vi "ColourElementTree(SubVI).vi"(8 "Error In":errorcluster, 9 "Color":u32(colorbox), 10 "SR Number":string, 11 "TreeControl in":refnum<vi>) -> (0 "Error Out":errorcluster)   [LabVIEW 2017, in "DS_Lib.lvlib" / "SRReportParser.lvlib"]
uses:
  SRReportParser.lvlib
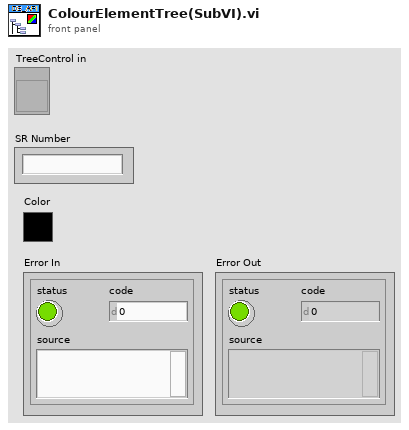
[diagram p1: front panel]
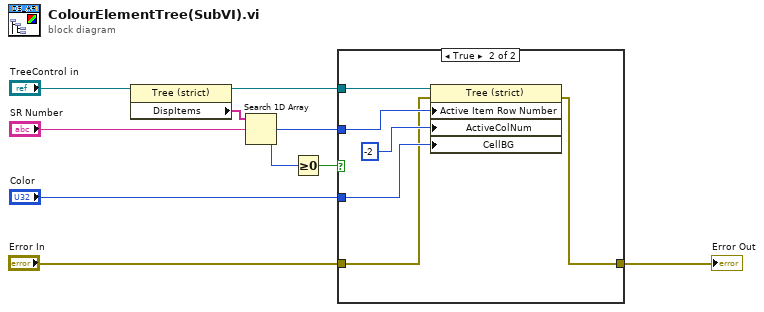
[diagram p0: block diagram]
diagram:
  n1 = property class="Tree (strict)"(reference="TreeControl in") -> (reference out=w9:refnum<vi>, "DispItems"=w8:string[])  [unwired: 1 in, 1 out]
  n2 = Search 1D Array(1D array=w8, element="SR Number") -> (index of element=w2:i32)  [unwired: 1 in]
  n3 = Greater Or Equal To 0?(x=w2) -> (x >= 0?=w1:bool)
  n4 = case shown="True" w1 {
    tunnel: w9 -> [_ w16]
    tunnel: w2 -> [_ w15]
    tunnel: "Color" -> [_ w13]
    tunnel: "Error In" -> [w10 w12]
    tunnel: [w10 w11] -> w3
    frame False {
    }
    frame True {
      n5 = property class="Tree (strict)"(reference=w16, error in=w12, "Active Item Row Number"=w15, "ActiveColNum"=-2 ("Active Cell:Active Column Number"), "CellBG"=w13) -> (error out=w11:errorcluster)  [unwired: 1 out]
    }
  }
  "Error Out" <- w3
